vi "RichToFlatniswitch_grpc_ScanRequest.vi"(5 "OutputClusterType":T1, 11 "InputCluster":T4) -> (3 "OutputCluster":T1)   [LabVIEW 2021, in "NI Switch_client.lvlib"]
uses:
  NI Switch_client.lvlib
  niswitch_grpc_ScanRequest.ctl
  niswitch_grpc_ScanRequest_initiation_enum/niswitch_grpc_ScanRequest_initiation_enum.lvclass
  nidevice_grpc_Session.ctl
  niswitch_grpc_ScanRequest_Flat.ctl
  nidevice_grpc_Session_Flat.ctl
  niswitch_grpc_HandshakingInitiation.ctl
  niswitch_grpc_ScanRequest_initiation_enum/niswitch_grpc_ScanRequest_initiation_enum.lvclass/niswitch_grpc_ScanRequest_initiation_enum.ctl
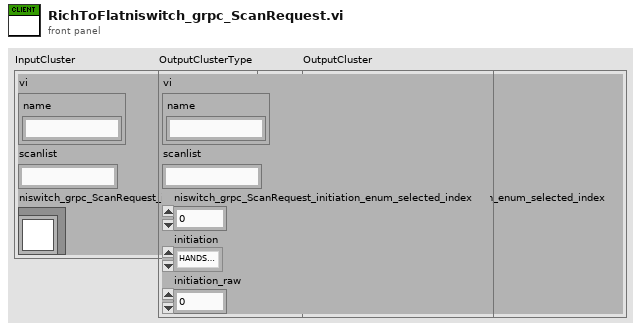
[diagram p1: front panel]
types:
  T1 = typedef "NI Switch_client.lvlib/niswitch_grpc_ScanRequest_Flat.ctl" = cluster{"vi":T2, "scanlist":string, "niswitch_grpc_ScanRequest_initiation_enum_selected_index":i32, "initiation":T3, "initiation_raw":i32}
  T2 = typedef "NI Switch_client.lvlib/nidevice_grpc_Session_Flat.ctl" = cluster{"name":string}
  T3 = typedef "NI Switch_client.lvlib/niswitch_grpc_HandshakingInitiation.ctl" = enum32{"HANDSHAKING_INITIATION_NISWITCH_VAL_MEASUREMENT_DEVICE_INITIATED", "HANDSHAKING_INITIATION_NISWITCH_VAL_SWITCH_INITIATED"}
  T4 = typedef "NI Switch_client.lvlib/niswitch_grpc_ScanRequest.ctl" = cluster{"vi":T5, "scanlist":string, "niswitch_grpc_ScanRequest_initiation_enum":refnum<class "niswitch_grpc_ScanRequest_initiation_enum.lvclass">}
  T5 = typedef "NI Switch_client.lvlib/nidevice_grpc_Session.ctl" = cluster{"name":string}
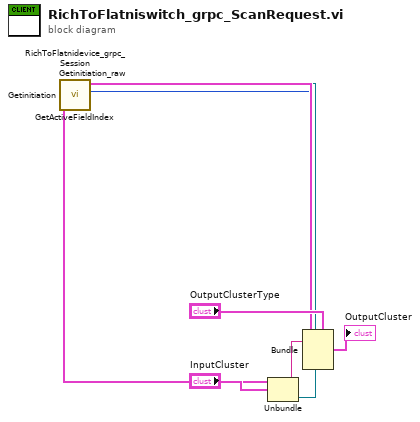
[diagram p0: block diagram]
diagram:
  n1 = Unbundle "Unbundle"("InputCluster") -> ("vi"=w7:T5, "scanlist"=w5:string, "niswitch_grpc_ScanRequest_initiation_enum"=w4:refnum<class "niswitch_grpc_ScanRequest_initiation_enum.lvclass">)
  n2 = call "Getinitiation_raw.vi"("OneOfTemplate in"=w4) -> ("Get_Val"=w1:i32)  [unwired: 8 in, 2 out]
  n3 = call "Getinitiation.vi"("OneOfTemplate in"=w4) -> ("Get_Val"=w2:T3)  [unwired: 8 in, 2 out]
  n4 = call "GetActiveFieldIndex.vi"("OneOfTemplate in"=w4) -> ("Active Field Index"=w3:i32)  [unwired: 8 in, 2 out]
  n5 = call "RichToFlatnidevice_grpc_Session.vi"("InputCluster"=w7) -> ("OutputCluster"=w6:T2)  [unwired: 10 in]
  n6 = Bundle "Bundle"(cluster="OutputClusterType", "vi"=w6, "scanlist"=w5, "niswitch_grpc_ScanRequest_initiation_enum_selected_index"=w3, "initiation"=w2, "initiation_raw"=w1) -> (→"OutputCluster":T1)
